vi "UpdateImg.vi"(7 "Enum":enum16{"Remove", "Mark", "Clear All"}(ring), 8 "error in (no error)":errorcluster, 11 "EpiWrapper in":refnum<class "EpiWrapper.lvclass">) -> (0 "error out":errorcluster, 3 "EpiWrapper out":refnum<class "EpiWrapper.lvclass">)   [LabVIEW 2012, in "EpiWrapper.lvclass"]
uses:
  EpiWrapper.lvclass
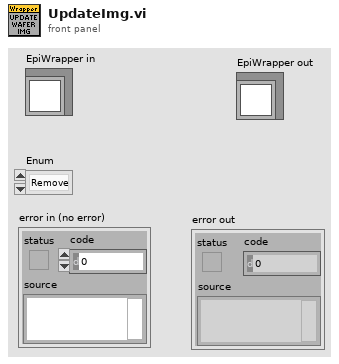
[diagram p1: front panel]
types:
  T1 = cluster{"Width":u16, "Style":enum32{"Solid", "Dash", "Dot", "DashDot", "DashDotDot"}}
  T2 = typedef "MapPOS.ctl" = cluster{"Coords":cluster{"Horizontal":sgl, "Vertical":sgl}, "radius":i32, "state":bool, "Id":string}[]
  T3 = typedef "SelectedPads.ctl" = T4[]
  T4 = typedef "Pad.ctl" = cluster{"Coords":cluster{"Horizontal":sgl, "Vertical":sgl}, "radius":i32, "Tested":bool, "Selected":bool, "Id":string}
  T5 = typedef "MeasureControl.ctl" = cluster{"Graph":cluster{"Y":dbl[], "Y":dbl[]}[], "Pass":bool, "Fail":bool, "Measure":bool, "Wafer Area":T6, "TestData":T7, "Pad":string}
  T6 = typedef "PadArea.ctl" = enum16{"A", "B", "C", "D", "L", "R", "T", "G"}
  T7 = typedef "TestData.ctl" = cluster{"20mA Data":T8, "50mA Data ":T8}
  T8 = typedef "Measurement.ctl" = cluster{"Area":string, "Pad":string, "Current,mA":dbl, "Power":dbl, "WL":dbl, "Voltage":dbl, "Knee Current":dbl, "Reverse":dbl}
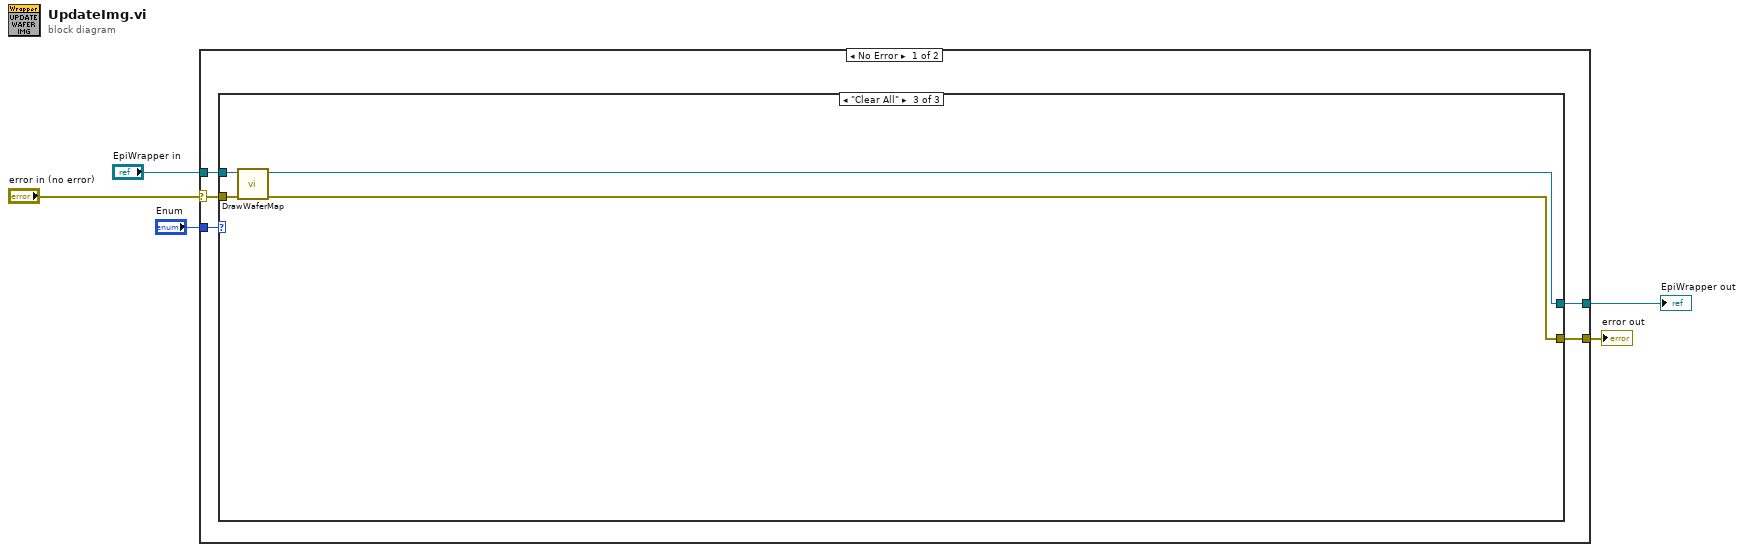
[diagram p0: block diagram]
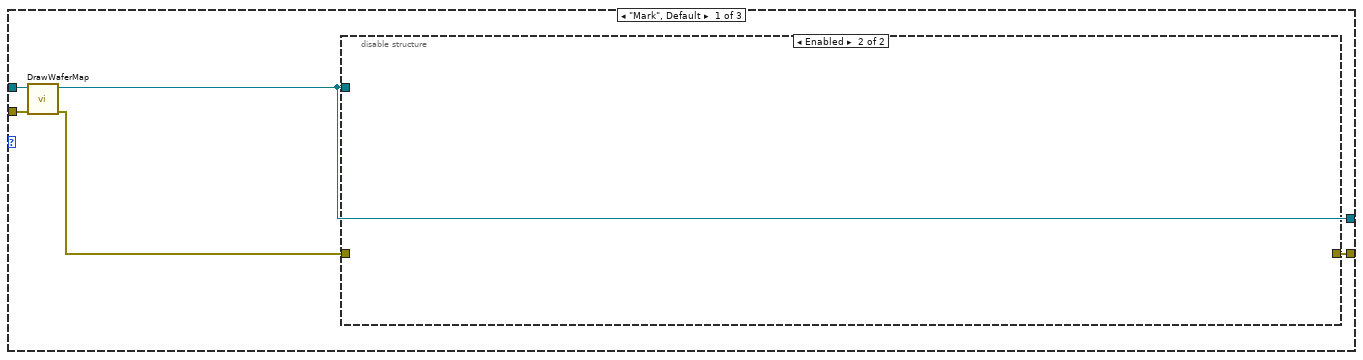
[diagram p2: hidden frame]
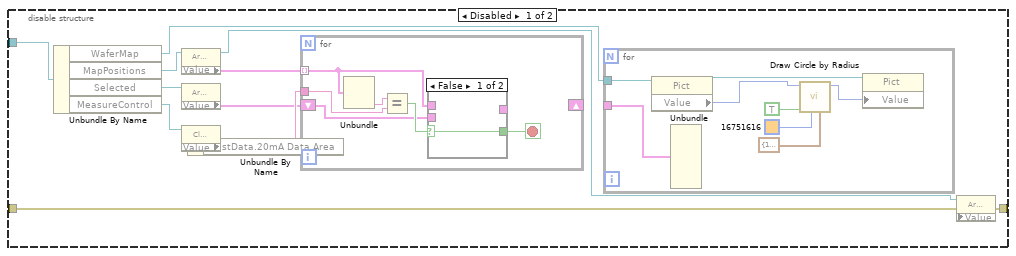
[diagram p3: hidden frame]
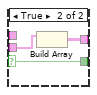
[diagram p4: hidden frame]
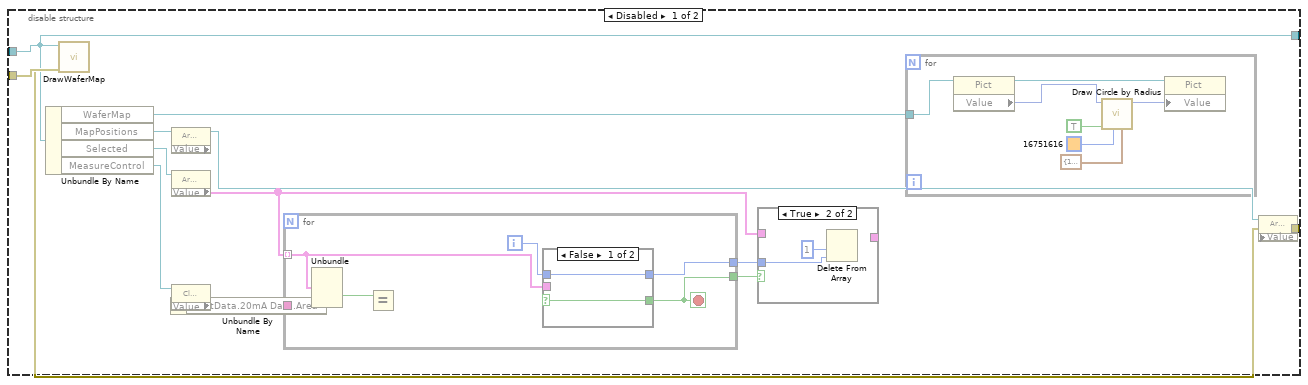
[diagram p6: hidden frame]
diagram:
  n1 = case shown="No Error" "error in (no error)" {
    selector: "error in (no error)" -> [w10 w90]
    tunnel: [w9 w90] -> w4
    tunnel: [w6 w89] -> w2
    tunnel: "EpiWrapper in" -> [w7 w89]
    tunnel: "Enum" -> [w8 _]
    frame No Error {
      n2 = case shown="\"Clear All\"" w8 {
        tunnel: w10 -> [w14 w48 w85]
        tunnel: [w12 w46 w86] -> w9
        tunnel: w7 -> [w15 w49 w88]
        tunnel: [w13 w47 w87] -> w6
        frame "Mark", Default {
          n3 = call-dynamic "DrawWaferMap.vi"("error in (no error)"=w14, "EpiWrapper in"=w15) -> ("error out"=w11:errorcluster, "EpiWrapper out"=w13:refnum<class "EpiWrapper.lvclass">)  [unwired: 8 in]
          n4 = disable-structure shown="Enabled" {
            disable-tunnel: w13 -> [w18 _]
            disable-tunnel: [w17 _] -> w12
            disable-tunnel: w11 -> [w16 _]
            frame Disabled {
              n5 = Unbundle By Name(w18) -> ("WaferMap"=w20:refnum<vi>, "MapPositions"=w23:refnum<vi>, "Selected"=w22:refnum<vi>, "MeasureControl"=w21:refnum<vi>)
              n6 = property class="Arr (strict)"(reference=w23) -> (reference out=w19:refnum<vi>, "Value"=w26:T2)  [unwired: 1 in, 1 out]
              n7 = property class="Arr (strict)"(reference=w22) -> ("Value"=w24:T3)  [unwired: 1 in, 2 out]
              n8 = property class="Clust (strict)"(reference=w21) -> ("Value"=w27:T5)  [unwired: 1 in, 2 out]
              n9 = Unbundle By Name(w27) -> ("TestData.20mA Data.Area"=w25:string)
              n10 = for {
                tunnel: w26 -> [w28] mode=indexing
                tunnel: w25 -> [w33]
                shift-right: _ -> [_]
                shift-left: w24 -> [w29]
                stop <- w30 stop-if-true
                n11 = Unbundle(w28) -> ("Id"=w32:string)  [unwired: 3 out]
                n12 = Equal?(x=w32, y=w33) -> (x = y?=w31:bool)
                n13 = case shown="False" w31 {
                  selector: w31 -> [w34 w37]
                  tunnel: [w34 w37] -> w30
                  tunnel: w29 -> [_ w36]
                  tunnel: w28 -> [_ _]
                  tunnel: [_ w35] -> _
                  frame False {
                  }
                  frame True {
                    n14 = Build Array(w36) -> (w35:T4[][])  [unwired: 1 in]
                  }
                }
              }
              n15 = for {
                tunnel: _ -> [w39]
                tunnel: w20 -> [w38]
                n16 = property class="Pict"(reference=w38) -> (reference out=w41:refnum<vi>, "Value"=w40:picture)  [unwired: 1 in, 1 out]
                n17 = Unbundle(w39) -> ()  [unwired: 8 out]
                n18 = call <vilib>:"Draw Circle by Radius.vi"("pen"=T1 {"Width"=1, "Style"=enum."Solid"}, "color(black)"=u32 16751616, "fill?(F)"=TRUE, "picture"=w40) -> ("new picture"=w42:picture)  [unwired: 7 in]
                n19 = property class="Pict"(reference=w41, "Value"=w42) -> ()  [unwired: 1 in, 2 out]
              }
              n20 = property class="Arr (strict)" props=["Value"](reference=w19, error in=w16) -> (error out=w17:errorcluster)  [unwired: 1 in, 1 out]
            }
            frame Enabled {
            }
          }
        }
        frame "Remove" {
          n21 = disable-structure shown="Enabled" {
            disable-tunnel: w49 -> [w62 w84]
            disable-tunnel: w48 -> [w61 _]
            disable-tunnel: [w56 w84] -> w47
            disable-tunnel: [w55 _] -> w46
            frame Disabled {
              n22 = call-dynamic "DrawWaferMap.vi"("error in (no error)"=w61, "EpiWrapper in"=w62) -> ("error out"=w54:errorcluster, "EpiWrapper out"=w56:refnum<class "EpiWrapper.lvclass">)  [unwired: 8 in]
              n23 = Unbundle By Name(w56) -> ("WaferMap"=w50:refnum<vi>, "MapPositions"=w60:refnum<vi>, "Selected"=w59:refnum<vi>, "MeasureControl"=w58:refnum<vi>)
              n24 = property class="Arr (strict)" props=["Value"](reference=w60) -> (reference out=w57:refnum<vi>)  [unwired: 1 in, 2 out]
              n25 = property class="Arr (strict)"(reference=w59) -> ("Value"=w51:T3)  [unwired: 1 in, 2 out]
              n26 = property class="Clust (strict)"(reference=w58) -> ("Value"=w64:T5)  [unwired: 1 in, 2 out]
              n27 = Unbundle By Name(w64) -> ("TestData.20mA Data.Area"=w63:string)
              n28 = for {
                tunnel: w51 -> [w78] mode=indexing
                tunnel: w63 -> [_]
                tunnel: [w77] -> w52
                tunnel: [w75] -> w53
                i -> [w76]
                stop <- w75 stop-if-true
                n29 = Unbundle(w78) -> ("Selected"=w79:bool)  [unwired: 4 out]
                n30 = Equal?(x=w79) -> ()  [unwired: 1 in, 1 out]
                n31 = case shown="False" {
                  selector: _ -> [w81 w83]
                  tunnel: [w81 w83] -> w75
                  tunnel: w78 -> [_ _]
                  tunnel: [w80 w82] -> w77
                  tunnel: w76 -> [w80 w82]
                  frame False {
                  }
                  frame True {
                  }
                }
              }
              n32 = case shown="True" w53 {
                tunnel: w52 -> [_ w74]
                tunnel: w51 -> [w72 _]
                tunnel: [w72 _] -> _
                frame False {
                }
                frame True {
                  n33 = Delete From Array(length=1, index=w74) -> ()  [unwired: 1 in, 2 out]
                }
              }
              n34 = for {
                tunnel: w50 -> [w65]
                n35 = property class="Pict"(reference=w65) -> (reference out=w67:refnum<vi>, "Value"=w66:picture)  [unwired: 1 in, 1 out]
                n36 = call <vilib>:"Draw Circle by Radius.vi"("pen"=T1 {"Width"=1, "Style"=enum."Solid"}, "color(black)"=u32 16751616, "fill?(F)"=TRUE, "picture"=w66) -> ("new picture"=w68:picture)  [unwired: 7 in]
                n37 = property class="Pict"(reference=w67, "Value"=w68) -> ()  [unwired: 1 in, 2 out]
              }
              n38 = property class="Arr (strict)" props=["Value"](reference=w57, error in=w54) -> (error out=w55:errorcluster)  [unwired: 1 in, 1 out]
            }
            frame Enabled {
            }
          }
        }
        frame "Clear All" {
          n39 = call-dynamic "DrawWaferMap.vi"("error in (no error)"=w85, "EpiWrapper in"=w88) -> ("error out"=w86:errorcluster, "EpiWrapper out"=w87:refnum<class "EpiWrapper.lvclass">)  [unwired: 8 in]
        }
      }
    }
    frame Error {
    }
  }
  "error out" <- w4
  "EpiWrapper out" <- w2
